vi "Set Print Speeds.vi"(8 "error in (no error)":errorcluster, 10 "Print Values":T1={"Screw"=1, "Inner"=0.0, "Outer"=0.0, "Mixer"=0.0} {"Mixer" scale=0.075..0.095; "Screw" items=["0%"=1, "25%"=225, "50%"=450, "75%"=675, "100%"=900]}, 11 "Main.lvlib:Main.lvclass":refnum<class "Main.lvclass">) -> (0 "error out":errorcluster, 3 "Main.lvlib:Main.lvclass 2":refnum<class "Main.lvclass">)   [LabVIEW 2018, in "Main.lvlib" / "Main.lvclass"]
uses:
  Main.lvclass
  Main.lvclass/Main.ctl
  MFC Actor/MFC Messages/Set Printing Flow Msg/Set Printing Flow Msg.lvclass/Set Printing Flow Msg.ctl
  <vilib>/ActorFramework/Message Enqueuer/Message Enqueuer.lvclass/Message Enqueuer.ctl
  <vilib>/ActorFramework/Message Enqueuer/Enqueue.vi
  MFC Actor/MFC Messages/Set Printing Flow Msg/Set Printing Flow Msg.lvclass
  C:/Program Files/National Instruments/LabVIEW 2018/vi.lib/ActorFramework/Message/Message.lvclass
  <vilib>/ActorFramework/Message Priority Queue/Priority Enqueue.vi
  Feeder Actor/Feeder Messages/Set Print Speeds Msg/Set Print Speeds Msg.lvclass
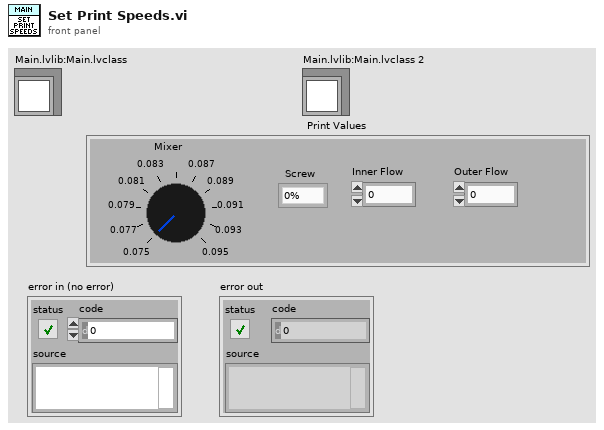
[diagram p1: front panel]
types:
  T1 = cluster{"Screw":u16, "Inner":dbl, "Outer":dbl, "Mixer":dbl}
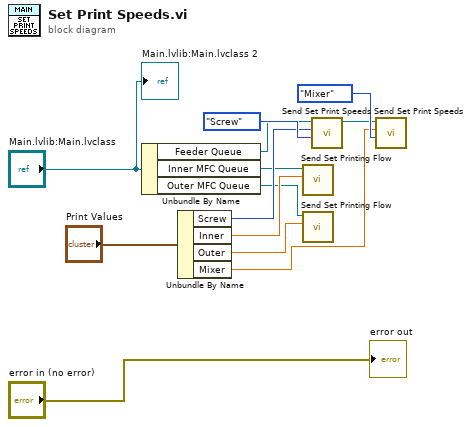
[diagram p0: block diagram]
diagram:
  n1 = Unbundle By Name("Main.lvlib:Main.lvclass") -> ("Feeder Queue"=w8:refnum<class "Message Enqueuer.lvclass">, "Inner MFC Queue"=w4:refnum<class "Message Enqueuer.lvclass">, "Outer MFC Queue"=w2:refnum<class "Message Enqueuer.lvclass">)
  n2 = Unbundle By Name("Print Values") -> ("Screw"=w9:u16, "Inner"=w5:dbl, "Outer"=w3:dbl, "Mixer"=w6:dbl)
  n3 = call "Send Set Printing Flow.vi"("Print Value"=w5, "Message Enqueuer in"=w4) -> ()  [unwired: 8 in, 2 out]
  n4 = call "Send Set Printing Flow.vi"("Print Value"=w3, "Message Enqueuer in"=w2) -> ()  [unwired: 8 in, 2 out]
  n5 = call "Send Set Print Speeds.vi"("Enum"=enum16{"Mixer", "Screw"}."Screw", "Speed"=w9, "Message Enqueuer in"=w8) -> ("Message Enqueuer out"=w7:refnum<class "Message Enqueuer.lvclass">)  [unwired: 7 in, 1 out]
  n6 = call "Send Set Print Speeds.vi"("Enum"=enum16{"Mixer", "Screw"}."Mixer", "Speed"=w6, "Message Enqueuer in"=w7) -> ()  [unwired: 7 in, 2 out]
  "Main.lvlib:Main.lvclass 2" <- "Main.lvlib:Main.lvclass"
  "error out" <- "error in (no error)"
